vi "Resize Panel.vi"(4 "panel height":i16, 6 "panel width":i16, 8 "error in":errorcluster {"code" format="%.0x"}, 11 "Panel":refnum<vi>) -> (0 "error out":errorcluster {"code" format="%.0x"}, 3 "Panel out":refnum<vi>)   [LabVIEW 2018, in "NISAST VI Scripting.lvlib" / "VI.lvlib" / "Front Panel.lvlib"]
uses:
  Front Panel.lvlib
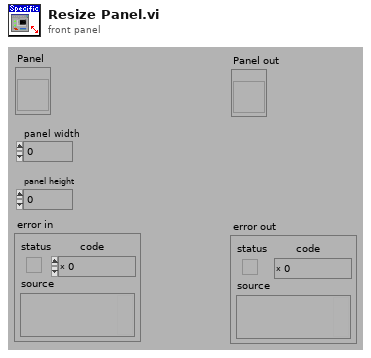
[diagram p1: front panel]
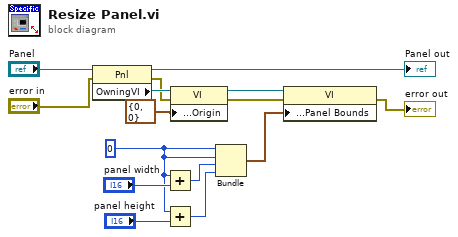
[diagram p0: block diagram]
diagram:
  w1 = i16 0 ("left")
  n1 = property class="Pnl"(reference="Panel", error in="error in") -> (reference out=→"Panel out":refnum<vi>, error out=w6:errorcluster, "OwningVI"=w9:refnum<vi>)
  n2 = Add(x=w1, y="panel width") -> (x+y=w4:i16)
  n3 = Add(x=w1, y="panel height") -> (x+y=w3:i16)
  n4 = property class="VI"(reference=w9, error in=w6, "Front Panel Window:Origin"=cluster{"Horizontal":i16, "Vertical":i16} {"Horizontal"=0, "Vertical"=0}) -> (reference out=w13:refnum<vi>, error out=w12:errorcluster)
  n5 = Bundle("left"=w1, "left"=w1, w4, w3) -> (w14:cluster{"left":i16, "left":i16, i16, i16})  [unwired: 1 out]
  n6 = property class="VI"(reference=w13, error in=w12, "Front Panel Window:Panel Bounds"=w14) -> (error out=→"error out":errorcluster)  [unwired: 1 out]
